vi "NaN Pad Data.vi"(9 "Measured":waveform(dbl)[](array[waveform]), 10 "dt(s)":dbl, 11 "Num dts elapsed":dbl) -> (3 "Array":waveform(dbl)[](array[waveform]))   [LabVIEW 2023, in "Instruments.lvlib" / "Instruments.lvclass"]
uses:
  Library/Instruments.lvclass
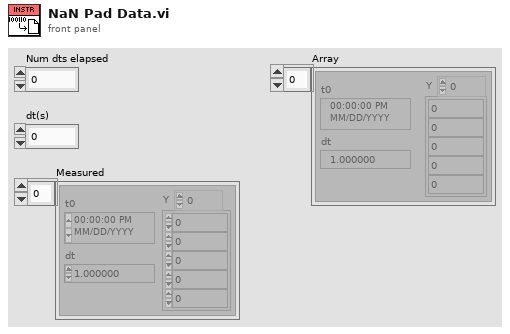
[diagram p1: front panel]
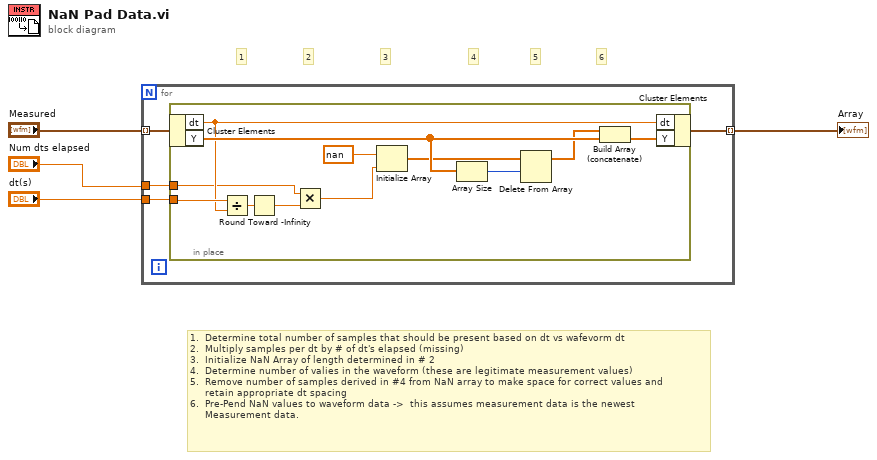
[diagram p0: block diagram]
diagram:
  # "1.  Determine total number of samples that should be present based on dt vs wafevorm dt\n2.  Multiply samples per dt by # of dt's elapsed (missing)\n3.  Initialize NaN Array of length determined in # 2\n4.  Determine number of valies in the waveform (these are legitimate measurement values)\n5.  Remove number of samples derived in #4 from NaN array to make space for correct values and \n     retain appropriate dt spacing\n6.  Pre-Pend NaN values to waveform data ->  this assumes measurement data is the newest \n     Measurement data."
  # "6"
  # "5"
  # "4"
  # "3"
  # "2"
  # "1"
  n1 = for {
    tunnel: "Measured" -> [w8] mode=indexing
    tunnel: [w7] -> w3 mode=indexing
    tunnel: "Num dts elapsed" -> [w5]
    tunnel: "dt(s)" -> [w6]
    n2 = in-place {
      in-place-border: w6 -> [w16]
      in-place-border: w5 -> [w11]
      n3 = in-place-cluster #1(w8) -> ("dt"=w15:dbl, "Y"=w20:dbl[])
      n4 = Divide(x=w16, y=w15) -> (x/y=w12:dbl)
      n5 = Round Toward -Infinity(1:w12) -> (0:w9:dbl)
      n6 = Multiply(x=w11, y=w9) -> (x*y=w10:dbl)
      n7 = Initialize Array(nan, w10) -> (w13:dbl[])
      n8 = Array Size(array=w20) -> (size(s)=w19:i32)
      n9 = Delete From Array(array=w13, length=w19) -> (array with subset deleted=w18:dbl[])  [unwired: 1 in, 1 out]
      n10 = Build Array (concatenate)(w18, w20) -> (w17:dbl[])
      n11 = in-place-cluster #1("dt"=w15, "Y"=w17) -> (w7:waveform(dbl))
    }
  }
  "Array" <- w3
